vi "4_2_spectral Leakage.vi"() -> ()   [LabVIEW 2009]
uses:
  <vilib>/Analysis/2dsp.llb/Real FFT.vi
  <vilib>/measure/matone.llb/Extract Single Tone Information 1 Chan.vi
  <vilib>/Analysis/NI_AALBase.lvlib
  <vilib>/measure/NI_MAPro.lvlib
  <vilib>/Analysis/NI_AALPro.lvlib
panel:
  out "FFT  SPEC.":dbl[](graph)=[6.53936540334632e-18, 5.2562522540870746e-18, 7.519706494921055e-18, 1.6919917446132515e-17, 4.221025736669126e-17, 0.5, 4.50258709793495e-17, 2.6497469438649404e-17, 1.7285828936833936e-17, 1.5351341060366622e-17, 6.8977519521584125e-18, 1.0057761539889605e-17, 9.302573231454864e-18, 5.3898390044030424e-18, 6.7547084329322e-18, 3.858014324716387e-17, 6.4913802696330046e-18, 3.477838529463856e-18, 7.36790606401202e-18, 3.929010783579174e-18, 7.34520083392793e-18, 5.340822099286018e-18, 1.6116958898396141e-18, 5.8010953140553794e-18, 4.464780312262639e-18, 1.9137676813604244e-17, 4.775971008534903e-18, 4.821312750942843e-18, 3.064809248315466e-18, 6.093838105106124e-18, 7.965074784886846e-18, 4.981663089074923e-18, 3.718409799106291e-18, 4.0036357495350966e-18, 7.25849982140764e-18, 1.2540738181757668e-17, 4.408715417720828e-18, 6.156957379911326e-18, 2.2282746154832354e-18, 3.866070665214115e-18, 6.453537080937604e-18, 8.81475160107701e-19, 6.386200271468706e-18, 2.527609942521086e-18, 2.8279690664189e-18, 1.0924625258850671e-17, 2.625853620063216e-18, 4.3707497006399826e-18, 1.9848865370971834e-18, 4.046025266010334e-18]
  out "Frequency Resolution":dbl=10.0 format="%#_6p"
  out "?":bool
  out "?":bool
  out "?":string="Sample"
  in  "stop":bool
  out "DETECTED FREQ":dbl=0.05 format="%.2p"
  out "1-SIDED FFT SPECTRUM":cluster{i32, dbl, dbl[]}(graph)={0, 10.0, [6.53936540334632e-18, 1.0512504508174149e-17, 1.503941298984211e-17, 3.383983489226503e-17, 8.442051473338252e-17, 1.0, 9.0051741958699e-17, 5.299493887729881e-17, 3.457165787366787e-17, 3.0702682120733244e-17, 1.3795503904316825e-17, 2.011552307977921e-17, 1.860514646290973e-17, 1.0779678008806085e-17, 1.35094168658644e-17, 7.716028649432774e-17, 1.2982760539266009e-17, 6.955677058927712e-18, 1.473581212802404e-17, 7.858021567158349e-18, 1.469040166785586e-17, 1.0681644198572037e-17, 3.2233917796792282e-18, 1.1602190628110759e-17, 8.929560624525278e-18, 3.827535362720849e-17, 9.551942017069806e-18, 9.642625501885686e-18, 6.129618496630932e-18, 1.2187676210212249e-17, 1.593014956977369e-17, 9.963326178149846e-18, 7.436819598212583e-18, 8.007271499070193e-18, 1.451699964281528e-17, 2.5081476363515335e-17, 8.817430835441656e-18, 1.2313914759822652e-17, 4.456549230966471e-18, 7.73214133042823e-18, 1.2907074161875208e-17, 1.762950320215402e-18, 1.2772400542937411e-17, 5.055219885042172e-18, 5.6559381328378e-18, 2.1849250517701342e-17, 5.251707240126432e-18, 8.741499401279965e-18, 3.969773074194367e-18, 8.092050532020667e-18]}
  out "# OF CYCLES":dbl=5.0
  in  "?":bool
  out "PERIODIC REPETITION":dbl[](graph)=[0.0, 0.3090169943749474, 0.5877852522924731, 0.8090169943749475, 0.9510565162951535, 1.0, 0.9510565162951535, 0.8090169943749475, 0.5877852522924731, 0.30901699437494745, 5.307169634316544e-17, -0.3090169943749474, -0.587785252292473, -0.8090169943749473, -0.9510565162951535, -1.0, -0.9510565162951536, -0.8090169943749475, -0.5877852522924732, -0.3090169943749475, -1.0614339268633088e-16, 0.30901699437494734, 0.587785252292473, 0.8090169943749473, 0.9510565162951535, 1.0, 0.9510565162951536, 0.8090169943749476, 0.5877852522924732, 0.30901699437494756, 1.5921508902949633e-16, -0.3090169943749473, -0.587785252292473, -0.8090169943749473, -0.9510565162951535, -1.0, -0.9510565162951536, -0.8090169943749476, -0.5877852522924732, -0.3090169943749476, -2.1228678537266177e-16, 0.30901699437494723, 0.5877852522924729, 0.8090169943749473, 0.9510565162951535, 1.0, 0.9510565162951536, 0.8090169943749476, 0.5877852522924734, 0.3090169943749477, 2.653584817158272e-16, -0.3090169943749472, -0.5877852522924729, -0.8090169943749472, -0.9510565162951535, -1.0, -0.9510565162951536, -0.8090169943749476, -0.5877852522924734, -0.30901699437494773, -3.1843017805899265e-16, 0.3090169943749471, 0.5877852522924729, 0.8090169943749472, 0.9510565162951534, 1.0, 0.9510565162951536, 0.8090169943749477, 0.5877852522924735, 0.3090169943749478, 3.715018744021581e-16, -0.30901699437494706, -0.5877852522924728, -0.8090169943749472, -0.9510565162951534, -1.0, -0.9510565162951536, -0.8090169943749477, -0.5877852522924735, -0.30901699437494784, -4.2457357074532354e-16, 0.309016994374947, 0.5877852522924728, 0.8090169943749471, 0.9510565162951534, 1.0, 0.9510565162951538, 0.8090169943749477, 0.5877852522924735, 0.3090169943749479, 4.77645267088489e-16, -0.30901699437494695, -0.5877852522924727, -0.8090169943749471, -0.9510565162951534, -1.0, -0.9510565162951538, -0.8090169943749477, -0.5877852522924736, -0.30901699437494795, 0.0, 0.3090169943749474, 0.5877852522924731, 0.8090169943749475, 0.9510565162951535, 1.0, 0.9510565162951535, 0.8090169943749475, 0.5877852522924731, 0.30901699437494745, 5.307169634316544e-17, -0.3090169943749474, -0.587785252292473, -0.8090169943749473, -0.9510565162951535, -1.0, -0.9510565162951536, -0.8090169943749475, -0.5877852522924732, -0.3090169943749475, -1.0614339268633088e-16, 0.30901699437494734, 0.587785252292473, 0.8090169943749473, 0.9510565162951535, 1.0, 0.9510565162951536, 0.8090169943749476, 0.5877852522924732, 0.30901699437494756, 1.5921508902949633e-16, -0.3090169943749473, -0.587785252292473, -0.8090169943749473, -0.9510565162951535, -1.0, -0.9510565162951536, -0.8090169943749476, -0.5877852522924732, -0.3090169943749476, -2.1228678537266177e-16, 0.30901699437494723, 0.5877852522924729, 0.8090169943749473, 0.9510565162951535, 1.0, 0.9510565162951536, 0.8090169943749476, 0.5877852522924734, 0.3090169943749477, 2.653584817158272e-16, -0.3090169943749472, -0.5877852522924729, -0.8090169943749472, -0.9510565162951535, -1.0, -0.9510565162951536, -0.8090169943749476, -0.5877852522924734, -0.30901699437494773, -3.1843017805899265e-16, 0.3090169943749471, 0.5877852522924729, 0.8090169943749472, 0.9510565162951534, 1.0, 0.9510565162951536, 0.8090169943749477, 0.5877852522924735, 0.3090169943749478, 3.715018744021581e-16, -0.30901699437494706, -0.5877852522924728, -0.8090169943749472, -0.9510565162951534, -1.0, -0.9510565162951536, -0.8090169943749477, -0.5877852522924735, -0.30901699437494784, -4.2457357074532354e-16, 0.309016994374947, 0.5877852522924728, 0.8090169943749471, 0.9510565162951534, 1.0, 0.9510565162951538, 0.8090169943749477, 0.5877852522924735, 0.3090169943749479, 4.77645267088489e-16, -0.30901699437494695, -0.5877852522924727, -0.8090169943749471, -0.9510565162951534, -1.0, -0.9510565162951538, -0.8090169943749477, -0.5877852522924736, -0.30901699437494795]
  in  "Delta t":dbl=0.1 format="%0.2f"
  in  "Duty cycle (%)":dbl=50.0 format="%0.2f"
  in  "Width":i32=1
  in  "Start":dbl format="%0.2f"
  in  "End":dbl=1.0 format="%0.2f"
  out "ORIGINAL SIGNAL":T1(graph)={0, "# OF SAMPLES"=1.0, "Sinc Pattern"=[0.0, 0.3090169943749474, 0.5877852522924731, 0.8090169943749475, 0.9510565162951535, 1.0, 0.9510565162951535, 0.8090169943749475, 0.5877852522924731, 0.30901699437494745, 5.307169634316544e-17, -0.3090169943749474, -0.587785252292473, -0.8090169943749473, -0.9510565162951535, -1.0, -0.9510565162951536, -0.8090169943749475, -0.5877852522924732, -0.3090169943749475, -1.0614339268633088e-16, 0.30901699437494734, 0.587785252292473, 0.8090169943749473, 0.9510565162951535, 1.0, 0.9510565162951536, 0.8090169943749476, 0.5877852522924732, 0.30901699437494756, 1.5921508902949633e-16, -0.3090169943749473, -0.587785252292473, -0.8090169943749473, -0.9510565162951535, -1.0, -0.9510565162951536, -0.8090169943749476, -0.5877852522924732, -0.3090169943749476, -2.1228678537266177e-16, 0.30901699437494723, 0.5877852522924729, 0.8090169943749473, 0.9510565162951535, 1.0, 0.9510565162951536, 0.8090169943749476, 0.5877852522924734, 0.3090169943749477, 2.653584817158272e-16, -0.3090169943749472, -0.5877852522924729, -0.8090169943749472, -0.9510565162951535, -1.0, -0.9510565162951536, -0.8090169943749476, -0.5877852522924734, -0.30901699437494773, -3.1843017805899265e-16, 0.3090169943749471, 0.5877852522924729, 0.8090169943749472, 0.9510565162951534, 1.0, 0.9510565162951536, 0.8090169943749477, 0.5877852522924735, 0.3090169943749478, 3.715018744021581e-16, -0.30901699437494706, -0.5877852522924728, -0.8090169943749472, -0.9510565162951534, -1.0, -0.9510565162951536, -0.8090169943749477, -0.5877852522924735, -0.30901699437494784, -4.2457357074532354e-16, 0.309016994374947, 0.5877852522924728, 0.8090169943749471, 0.9510565162951534, 1.0, 0.9510565162951538, 0.8090169943749477, 0.5877852522924735, 0.3090169943749479, 4.77645267088489e-16, -0.30901699437494695, -0.5877852522924727, -0.8090169943749471, -0.9510565162951534, -1.0, -0.9510565162951538, -0.8090169943749477, -0.5877852522924736, -0.30901699437494795]}
  in  "Reset phase":bool=TRUE
  in  "DELAY":dbl(knob) min=0.0 max=10.0 scale=0.0..10.0
  in  "SAMPLING\nFREQUENCY (Hz)":dbl(slide)=1000.0 scale=0.0..50000.0 scale format="%#_6p"
  in  "# OF SAMPLES (N)":dbl=100.0
  in  "AMPLITUDE":dbl=1.0
  in  "PHASE IN":dbl(knob) scale=0.0..180.0
  in  "SIGNAL FREQUENCY":dbl(knob)=50.0 scale=0.0..10000.0 scale format="%#_6p"
  in  "SIGNAL":T2(ring)
  # "Program developed by Indranil Sinharoy"
  # "SAMPLING INFO"
  # "ORIGINAL SIGNAL \nCHARACTERISTICS"
  # "RAMP"
  # "PULSE"
  # "SQUARE"
  # "SINC"
  # "X[k]"
  # "(Fundamental Freq)"
  # "fanalysis (k) = kfs/N, where k = 0,1,2,3,.......,N-1. \nThe DFT produces correct results only when the input data sequence contains energy precisely at the analysis frequencies, at integral multiples of fundamental frequency fs/N.\nIf the input has a signal component at some intermediate frequency between the analytical frequencies of kfs/N, this input signal will show up to some degree in all of the N output analysis frequencies of the DFT spectrum."
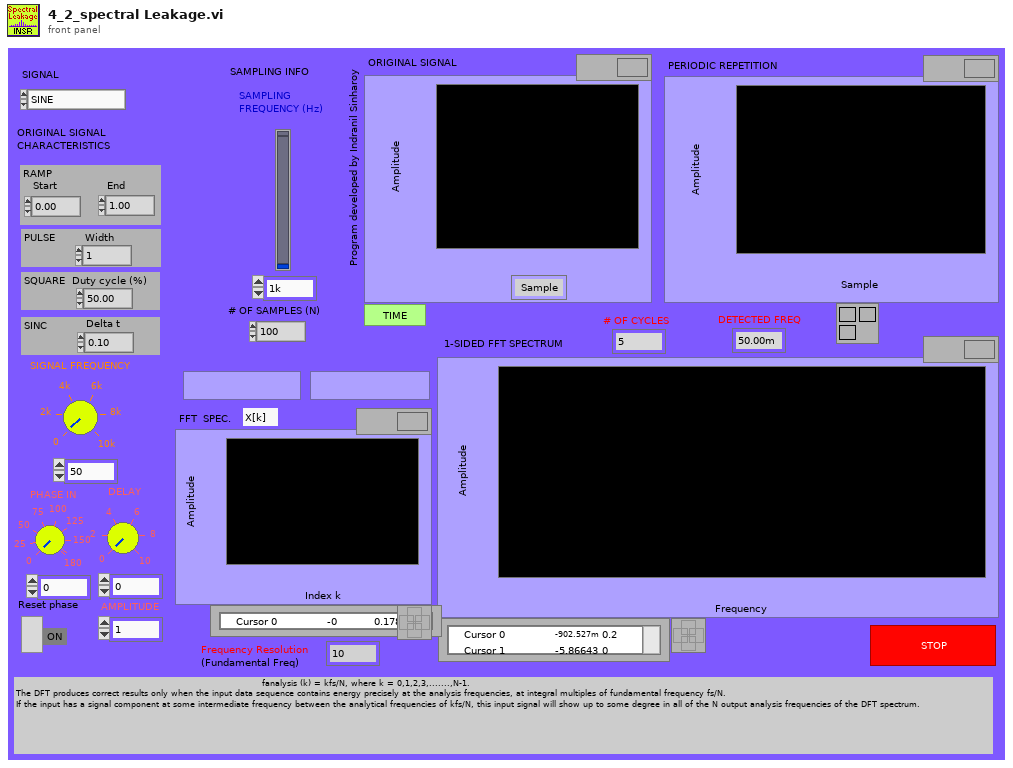
[diagram p1: front panel]
types:
  T1 = cluster{i32, "# OF SAMPLES":dbl, "Sinc Pattern":dbl[]}
  T2 = enum16{"SINE", "TRIANGULAR", "RAMP", "IMPULSE", "SINC ", "PULSE", "SQUARE"}
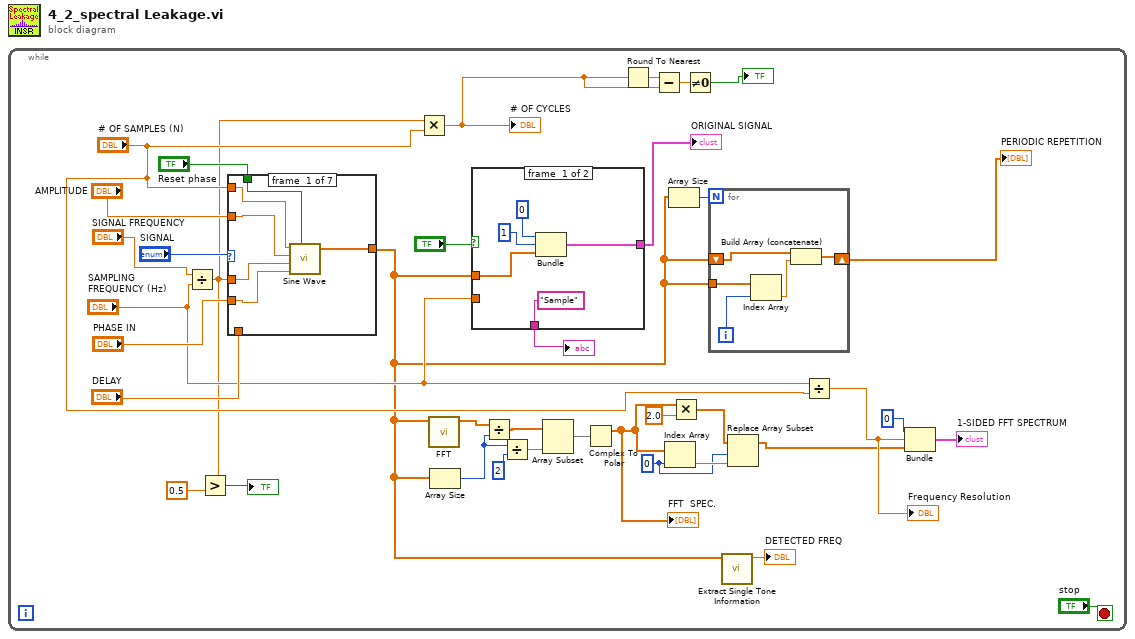
[diagram p0: block diagram]
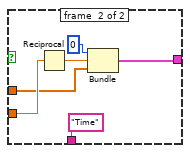
[diagram p2: hidden frame]
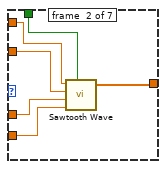
[diagram p3: hidden frame]
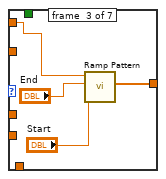
[diagram p4: hidden frame]
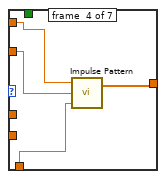
[diagram p5: hidden frame]
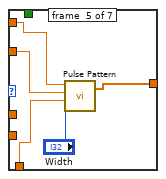
[diagram p6: hidden frame]
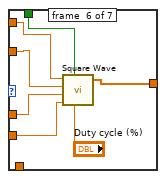
[diagram p7: hidden frame]
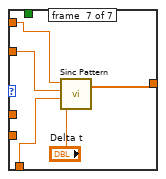
[diagram p8: hidden frame]
diagram:
  n1 = while {
    stop <- "stop" stop-if-true
    w22 = 0 ("index")
    n2 = Divide(x="SIGNAL FREQUENCY", y="SAMPLING\nFREQUENCY (Hz)") -> (x/y=w10:dbl)
    n3 = Greater?(x=w10, y=0.5) -> (0:→"?":bool)
    n4 = case shown="\"RAMP\"" "SIGNAL" {
      tunnel: "Reset phase" -> [w60 w66 _ _ _ w86 _]
      tunnel: "AMPLITUDE" -> [w58 w64 _ w73 w78 w84 w90]
      tunnel: "# OF SAMPLES (N)" -> [w59 w65 w69 w74 w79 w85 w91]
      tunnel: w10 -> [w57 w63 _ _ _ w83 _]
      tunnel: "PHASE IN" -> [w56 w62 _ _ _ w82 _]
      tunnel: "DELAY" -> [_ _ _ w72 w77 _ w89]
      tunnel: [w55 w61 w70 w71 w76 w81 w88] -> w16
      frame #0 {
        n5 = call <vilib>:"Sine Wave.vi"("samples"=w59, "amplitude"=w58, "frequency"=w57, "phase in"=w56, "reset phase"=w60) -> ("sine wave"=w55:dbl[])  [unwired: 2 out]
      }
      frame #1 {
        n6 = call <vilib>:"Sawtooth Wave.vi"("samples"=w65, "amplitude"=w64, "frequency"=w63, "phase in"=w62, "reset phase"=w66) -> ("sawtooth wave"=w61:dbl[])  [unwired: 2 out]
      }
      frame #2 {
        n7 = call <vilib>:"Ramp Pattern.vi"("start"="Start", "end"="End", "samples"=w69) -> ("Ramp Pattern"=w70:dbl[])  [unwired: 7 in, 1 out]
      }
      frame #3 {
        n8 = call <vilib>:"Impulse Pattern.vi"("delay"=w72, "amplitude"=w73, "samples"=w74) -> ("Impulse Pattern"=w71:dbl[])  [unwired: 1 out]
      }
      frame #4 {
        n9 = call <vilib>:"Pulse Pattern.vi"("width"="Width", "delay"=w77, "amplitude"=w78, "samples"=w79) -> ("Pulse Pattern"=w76:dbl[])  [unwired: 1 out]
      }
      frame #5 {
        n10 = call <vilib>:"Square Wave.vi"("samples"=w85, "reset phase"=w86, "amplitude"=w84, "frequency"=w83, "duty cycle (%)"="Duty cycle (%)", "phase in"=w82) -> ("square wave"=w81:dbl[])  [unwired: 2 out]
      }
      frame #6 {
        n11 = call <vilib>:"Sinc Pattern.vi"("delta t"="Delta t", "delay"=w89, "amplitude"=w90, "samples"=w91) -> ("Sinc Pattern"=w88:dbl[])  [unwired: 1 out]
      }
    }
    n12 = Multiply(x=w10, y="# OF SAMPLES (N)") -> (x*y=w7:dbl)
    "# OF CYCLES" <- w7
    n13 = call-poly <vilib>:"FFT.vi"("X"=w16) -> ("FFT {X}"=w29:cdb[])  [unwired: 9 in, 1 out]
    n14 = Array Size(array=w16) -> (size(s)=w26:i32)
    n15 = case shown="True" "?" {
      tunnel: w16 -> [w47 w52]
      tunnel: [w45 w50] -> w31
      tunnel: "SAMPLING\nFREQUENCY (Hz)" -> [_ w54]
      tunnel: ["Sample" "Time"] -> w12
      frame #0 {
        n16 = Bundle(0, 1, "Sinc Pattern"=w47) -> (w45:cluster{i32, i32, "Sinc Pattern":dbl[]})  [unwired: 1 in]
      }
      frame #1 {
        n17 = Reciprocal(x=w54) -> (1/x=w53:dbl)
        n18 = Bundle(0, w53, "Sinc Pattern"=w52) -> (w50:cluster{i32, dbl, "Sinc Pattern":dbl[]})  [unwired: 1 in]
      }
    }
    "ORIGINAL SIGNAL" <- w31
    "?" <- w12
    n19 = Divide(x=w29, y=w26) -> (x/y=w28:cdb[])
    n20 = Divide(x=w26, y=2) -> (x/y=w27:dbl)
    n21 = Array Subset(array=w28, length=w27) -> (w24:cdb[])  [unwired: 1 in]
    n22 = Complex To Polar(r * e^(i*theta)=w24) -> (r=w1:dbl[])  [unwired: 1 out]
    "FFT  SPEC." <- w1
    n23 = Round To Nearest(number=w7) -> (nearest integer value=w8:dbl)
    n24 = Subtract(x=w8, y=w7) -> (x-y=w6:dbl)
    n25 = Index Array(array=w1, index=w22) -> (element=w23:dbl)
    n26 = Array Size(array=w16) -> (size(s)=w30:i32)
    n27 = Multiply(x=w1, y=2.0) -> (x*y=w21:dbl[])
    n28 = Not Equal To 0?(x=w6) -> (x != 0?=→"?":bool)
    n29 = for {
      N: w30 -> [_]
      shift-right: [w42] -> w13
      shift-left: w16 -> [w41]
      tunnel: w16 -> [w39]
      i -> [w40]
      n30 = Index Array(array=w39, index=w40) -> (element=w43:dbl)
      n31 = Build Array (concatenate)(w41, w43) -> (w42:dbl[])
    }
    "PERIODIC REPETITION" <- w13
    n32 = call-poly <vilib>:"Extract Single Tone Information.vi"("time signal in"=w16) -> ("detected frequency"=→"DETECTED FREQ":dbl)  [unwired: 5 in, 5 out]
    n33 = Replace Array Subset(array=w21, new element=w23, index=w22) -> (w3:dbl[])
    n34 = Divide(x="SAMPLING\nFREQUENCY (Hz)", y="# OF SAMPLES (N)") -> (x/y=w4:dbl)
    "Frequency Resolution" <- w4
    n35 = Bundle(0, w4, w3) -> (→"1-SIDED FFT SPECTRUM":cluster{i32, dbl, dbl[]})  [unwired: 1 in]
  }
